vi "FPGAmain.vi"() -> ()   [LabVIEW 2013]
uses:
  FPGA/DataMode.ctl
  FPGA/AcquireState.ctl
  <vilib>/Platform/TimedLoop/XDataNode/timing_clust.ctl
  <vilib>/Platform/TimedLoop/XDataNode/nitl_modes.ctl
  <vilib>/Platform/TimedLoop/XDataNode/wakeup.ctl
  <vilib>/rvi/Emulation/niFpgaSctlEmulationGetInTimedLoop.vi
  <vilib>/rvi/Emulation/niFpgaEmulationReportErrorSimple.vi
  <vilib>/rvi/Emulation/niFpgaGetClockAttributes.vi
  <vilib>/rvi/Emulation/niFpgaCriticalErrorInLSC.vi
  <vilib>/rvi/FIFO/Fifo_Resource/nirvififoEmulationWriteFpgaImpl.vi
  <vilib>/rvi/DataTransferAndStorage/Container/Common/niFpgaContainerGetUniqueNameForEmu.vi
  <vilib>/rvi/FIFO/Fifo_Resource/nirvififoEmulationReadFpgaImpl.vi
  <vilib>/rvi/interface/RandomDataEmulation/nirviRandomDataMultiElementFPGAFIFO.vi
  <instcachedir>/0/nirviRandomDataMultiElementFPGAFIFO_F2B80EDE0D7944A08478D8D26097D4DB.lvgen/nirviRandomDataMultiElementFPGAFIFO_F2B80EDE0D7944A08478D8D26097D4DB_005.vi
  <vilib>/rvi/interface/RandomDataEmulation/niFpgaRandomDataHandleErrors.vi
  <vilib>/rvi/interface/RandomDataEmulation/nirviRandomDataFPGAFIFO.vi
  <vilib>/rvi/eio/common/nirviEmuTemplateMethod_errors.vi
  <vilib>/Platform/TimedLoop/XDataNode/XDataNode.xnode
  <vilib>/rvi/DataTransferAndStorage/Container/XNode/niFpgaContainer.xnode
  <vilib>/rvi/FIFO/Fifo_Resource/nirvififoEmulationWrite.vi
  <vilib>/rvi/FIFO/Fifo_Resource/nirvififoEmulationRead.vi
  <vilib>/rvi/interface/RandomDataEmulation/nirviRandomDataFpgaMultiElementTemplate.vi
  <vilib>/rvi/interface/RandomDataEmulation/nirviRandomDataFpgaReadWriteTemplate.vi
  <vilib>/eio/EIONode/EIONode.xnode
  <vilib>/rvi/FIFO/Fifo_Resource/nirvififoEmulationP2P.vi
  <vilib>/Platform/TimedLoop/XDataNode/XDNodeRunTimeDep.lvlib
  <instrlib>/FlexRIO/Libraries/Helper VIs/NI FlexRIO Helper VIs.lvlib
panel:
  in  "CIC Gain":fxp<+/-,32,1>=0.00390625 format="%#_32g"
  in  "Set downsample":bool
  in  "FIR coeffs":fxp<+/-,18,18>[](array[numeric])
  in  "FIR shift":i32
  in  "new coeffs":bool
  in  "enable filter":bool
  in  "Downsample":fxp<+,8,8>
  in  "Samples Per Trigger":i32 min=1 step=1
  in  "Trigger simulated data":bool
  in  "simulated phase 51600":fxp<+,64,64>
  in  "phase 5160":fxp<+,64,64>
  in  "Simulated phase 5772":fxp<+,64,64>[](array[numeric])=[0.0, 0.0, 0.0, 0.0]
  in  "Mode":T1
  in  "Phase 5772":fxp<+,64,64>[](array[numeric])=[0.0, 0.0, 0.0, 0.0]
  in  "Acquisition running":bool
  in  "User Command Commit":bool
  in  "User Command":u8
  out "User Command Idle":bool
  out "User Command Status":u8
  in  "User Data 0":u16
  in  "User Data 1":u8
  out "PLL Locked":bool
  out "User Error":bool
  out "Configured?":bool
  # "Dynamic filter"
  # "Dynamic downsample"
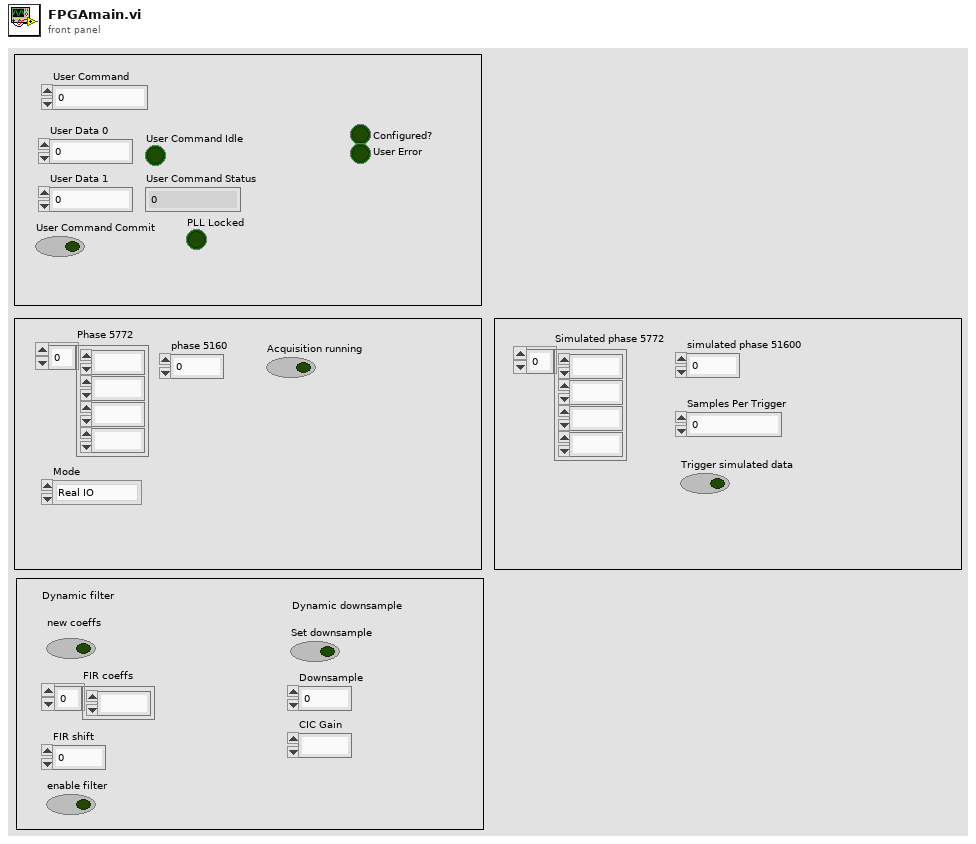
[diagram p1: front panel]
types:
  T1 = typedef "DataMode.ctl" = enum16{"Real IO", "Simulated"}
  T2 = typedef "AcquireState.ctl" = enum8{"Idle", "Acquire"}
  T3 = typedef "XDNodeRunTimeDep.lvlib/timing_clust.ctl" = cluster{"Expected End [f-1]":u64, "Actual End [f-1]":u64, "Finished Late? [f-1]":bool, "Expected End [i-1]":u64, "Actual End [i-1]":u64, "Finished Late? [i-1]":bool, "Expected Start [i]":u64, "Actual Start [i]":u64, "Expected Start [f]":u64, "Actual Start [f]":u64, "Source Name":string, "Structure Name":string, "Period":i64, "Deadline":i64, "Offset":i64, "Start":i64, "Priority":i32, "Timeout":i32, "Mode":T4, "Wakeup Reason":T5, "Error":errorcluster, "Source Type":string, "Secondary Source Type":string, "Global End Time":u64, "Global Start Time":u64, "Frame Duration":u64, "Iteration Duration":u64, "Assigned CPU":i32, "I/O Scan Engine Mode":u32}
  T4 = typedef "XDNodeRunTimeDep.lvlib/nitl_modes.ctl" = enum32{"No Change", "Process missed periods, maintain original phase", "Discard missed periods, maintain original phase", "Process missed periods, ignore original phase", "Discard missed periods, ignore original phase"}
  T5 = typedef "XDNodeRunTimeDep.lvlib/wakeup.ctl" = enum32{"Normal", "Aborted", "Asynchronous wakeup", "Timing source error", "Timed loop error", "Timeout"}
  T6 = typedef "I16 array size 4.ctl" = i16[]
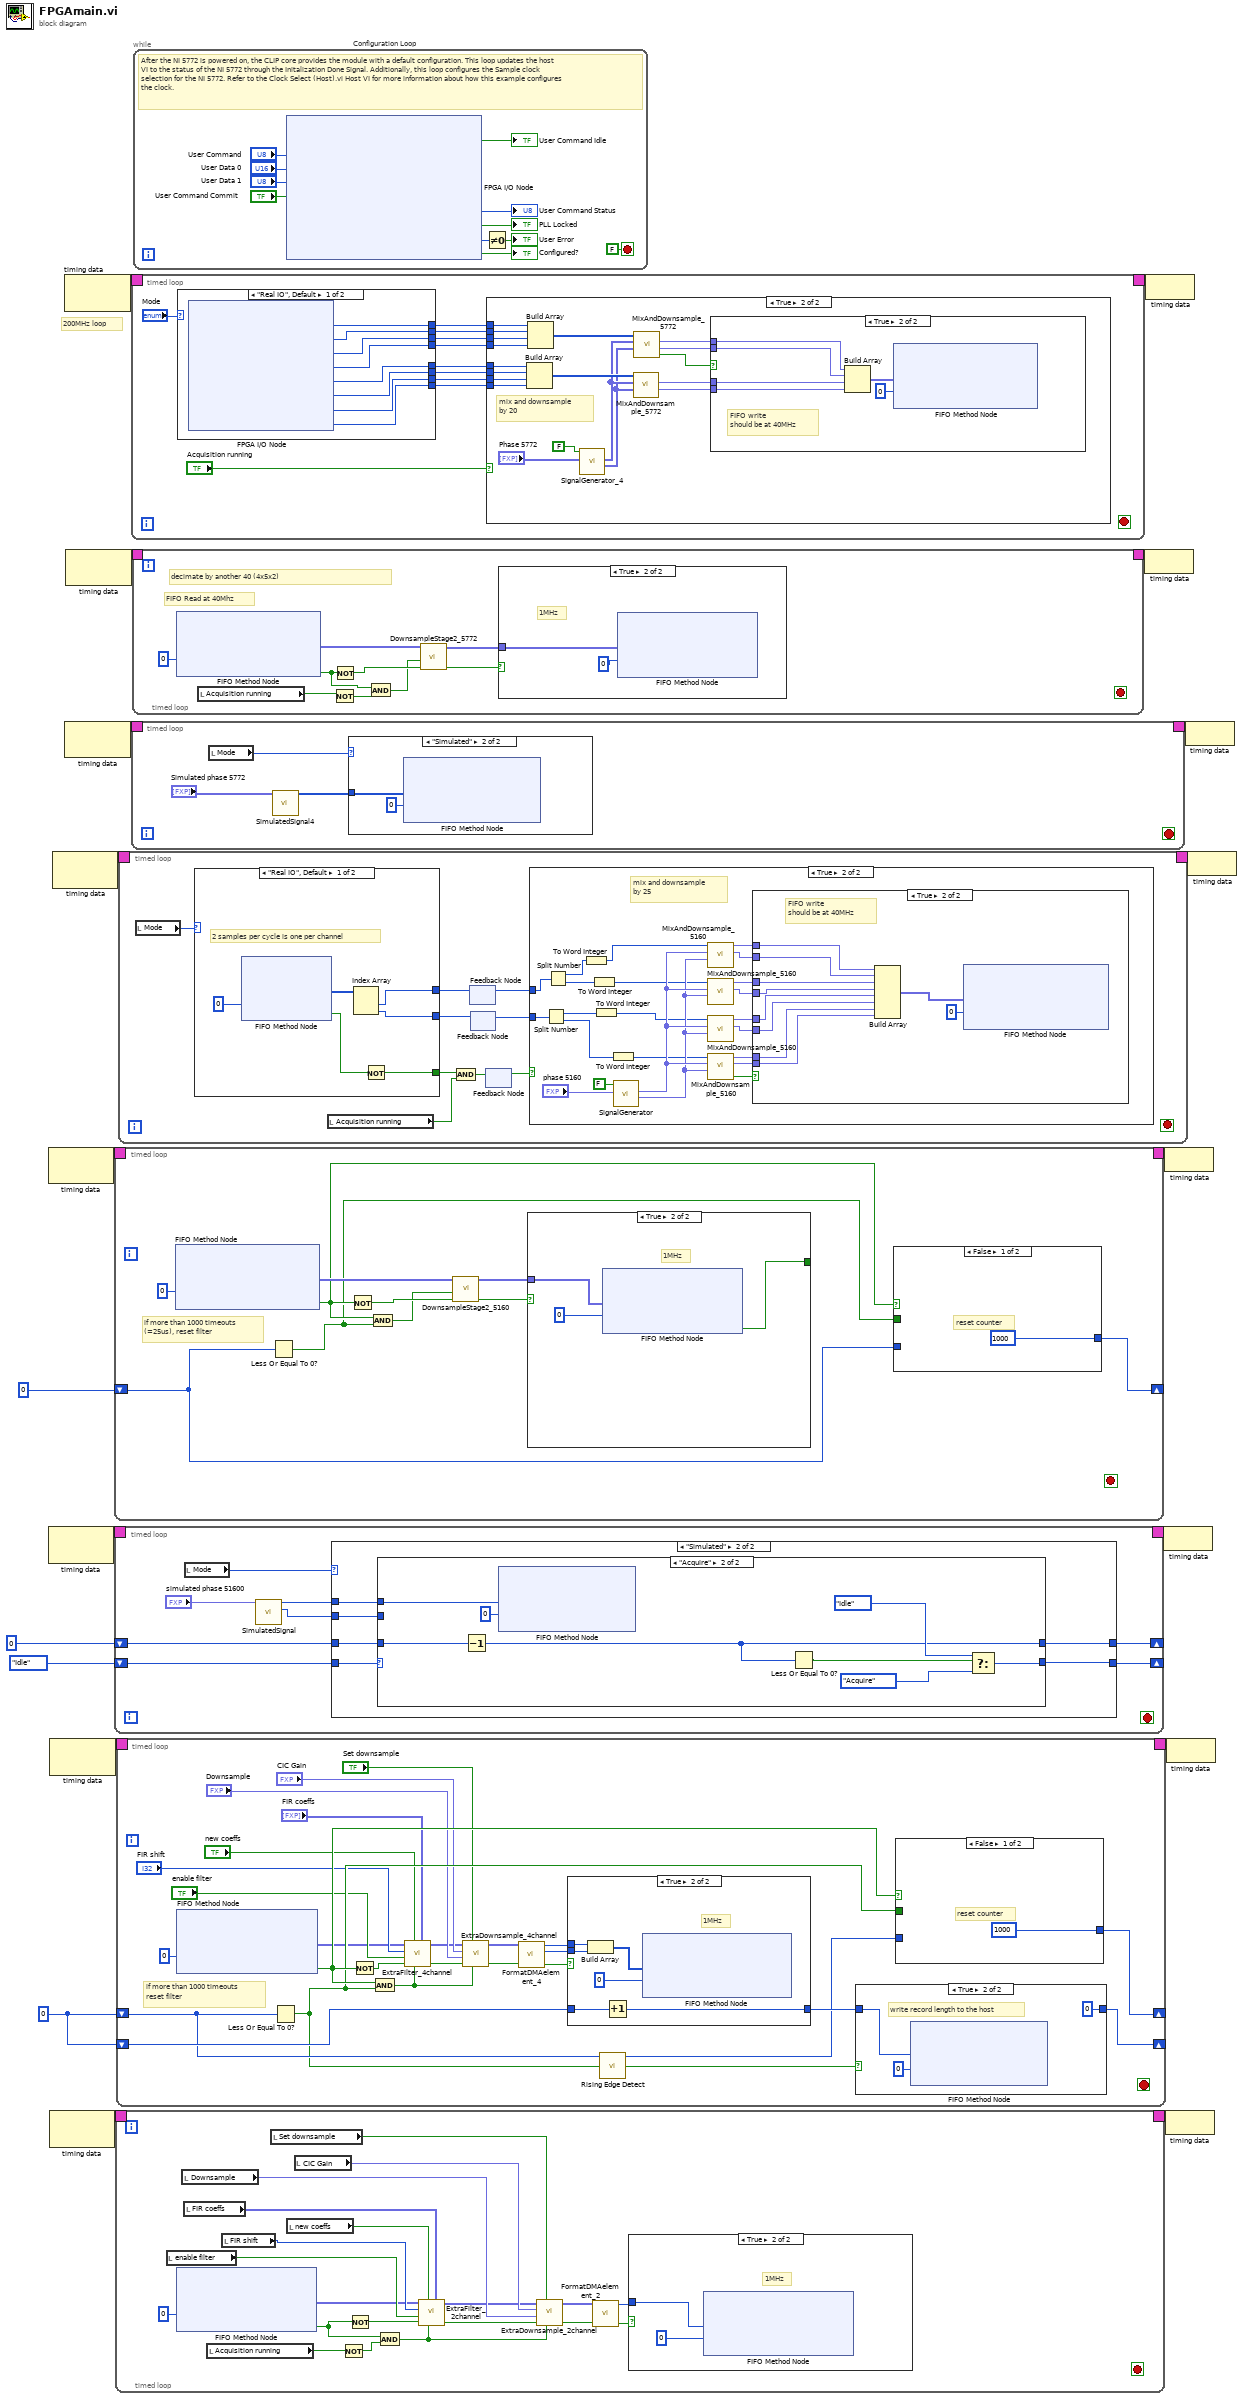
[diagram p0: block diagram]
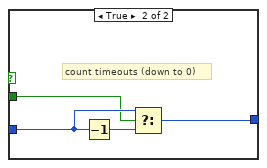
[diagram p3: hidden frame]
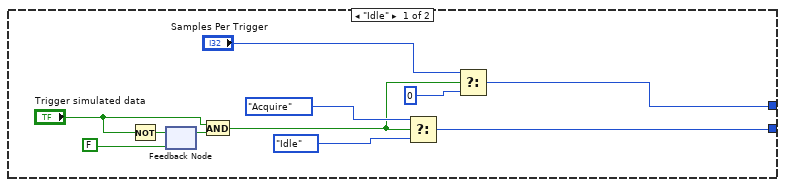
[diagram p7: hidden frame]
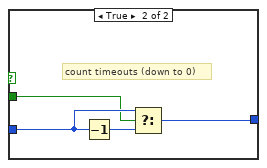
[diagram p8: hidden frame]
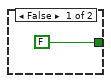
[diagram p9: hidden frame]
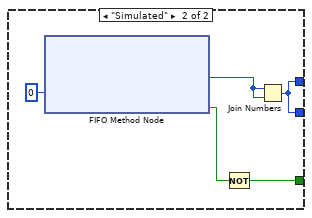
[diagram p12: hidden frame]
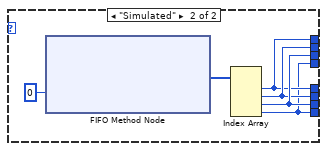
[diagram p17: hidden frame]
diagram:
  w1 = 0 ("y")
  # "200MHz loop"
  n1 = node-c288() -> (w12:T3)  [unwired: 1 in]
  n2 = node-c288() -> (w10:T3)  [unwired: 1 in]
  n3 = node-c288() -> (w3:T3)  [unwired: 1 in]
  n4 = node-c288() -> (w5:T3)  [unwired: 1 in]
  n5 = node-c288() -> (w14:T3)  [unwired: 1 in]
  n6 = node-c288() -> (w20:T3)  [unwired: 1 in]
  n7 = node-c288() -> (w16:T3)  [unwired: 1 in]
  n8 = node-c288() -> (w18:T3)  [unwired: 1 in]
  n9 = timed-loop {
    timing: w12 -> [_]
    timing-out: [_] -> w11
    shift-right: [w23] -> _
    shift-left: 0 ("y") -> [w22]
    stop <- _ stop-if-true
    # "if more than 1000 timeouts\n(=25us), reset filter"
    n10 = xnode ("FIFO Method Node")("Timeout"=0) -> ("Element"=w27:fxp<+/-,16,14>[], "Timed Out?"=w24:bool)  [unwired: 1 in, 1 out]
    n11 = Less Or Equal To 0?(x=w22) -> (x <= 0?=w21:bool)
    n12 = Not(x=w24) -> (.not. x?=w28:bool)
    n13 = And(x=w24, y=w21) -> (x .and. y?=w25:bool)
    n14 = call "DownsampleStage2_5160.vi"("valid in"=w28, "reset"=w25, "Element"=w27) -> ("valid out"=w29:bool, "Array"=w30:fxp<+/-,16,14>[])  [unwired: 7 in]
    n15 = case shown="True" w29 {
      tunnel: w30 -> [_ w37]
      tunnel: [FALSE ("Timed Out?") w38] -> _
      frame False {
      }
      frame True {
        # "1MHz"
        n16 = xnode ("FIFO Method Node")("Element"=w37, "Timeout"=0) -> ("Timed Out?"=w38:bool)  [unwired: 1 in, 1 out]
      }
    }
    n17 = case shown="False" w24 {
      tunnel: w21 -> [_ w33]
      tunnel: w22 -> [_ w34]
      tunnel: [1000 ("y") w32] -> w23
      frame False {
        # "reset counter"
      }
      frame True {
        # "count timeouts (down to 0)"
        n18 = Decrement(x=w34) -> (x-1=w35:i32)
        n19 = Select(t=w34, s=w33, f=w35) -> (s? t:f=w32:i32)
      }
    }
  }
  n20 = timed-loop {
    timing: w10 -> [_]
    timing-out: [_] -> w9
    shift-right: [w45] -> _
    shift-left: 0 ("f") -> [w44]
    shift-right: [w43] -> _
    shift-left: AcquireState."Idle" ("Acquire State") -> [w42]
    stop <- _ stop-if-true
    n21 = local read "Mode"() -> (w49:T1)
    n22 = call "SimulatedSignal.vi"("phase"="simulated phase 51600") -> ("cos output"=w47:i16, "Sample output"=w48:i16)  [unwired: 9 in]
    n23 = case shown="\"Simulated\"" w49 {
      tunnel: w48 -> [_ w57]
      tunnel: w47 -> [_ w52]
      tunnel: [w51 w56] -> w45
      tunnel: w44 -> [w51 w55]
      tunnel: [w50 w54] -> w43
      tunnel: w42 -> [w50 w53]
      frame "Real IO" {
      }
      frame "Simulated" {
        n24 = case shown="\"Acquire\"" w53 {
          tunnel: w55 -> [_ w73]
          tunnel: [w62 w72] -> w54
          tunnel: [w59 w71] -> w56
          tunnel: w57 -> [_ w70]
          tunnel: w52 -> [_ _]
          frame "Idle" {
            n25 = Not(x="Trigger simulated data") -> (.not. x?=w63:bool)
            n26 = feedback #1(FALSE) -> (w64:bool)
            n27 = feedback-in #1(w63) -> ()
            n28 = And(x="Trigger simulated data", y=w64) -> (x .and. y?=w58:bool)
            n29 = Select(t=AcquireState."Acquire" ("Acquire State"), s=w58, f=AcquireState."Idle" ("Acquire State")) -> (s? t:f=w62:T2)
            n30 = Select(t="Samples Per Trigger", s=w58, f=0) -> (s? t:f=w59:i32)
          }
          frame "Acquire" {
            n31 = Decrement(x=w73) -> (x-1=w71:i32)
            n32 = xnode ("FIFO Method Node")("Element"=w70, "Timeout"=0) -> ()  [unwired: 1 in, 2 out]
            n33 = Less Or Equal To 0?(x=w71) -> (x <= 0?=w75:bool)
            n34 = Select(t=AcquireState."Idle" ("Acquire State"), s=w75, f=AcquireState."Acquire" ("Acquire State")) -> (s? t:f=w72:T2)
          }
        }
      }
    }
  }
  n35 = timed-loop {
    timing: w3 -> [_]
    timing-out: [_] -> w2
    stop <- _ stop-if-true
    n36 = local read "enable filter"() -> (w94:bool)
    n37 = xnode ("FIFO Method Node")("Timeout"=0) -> ("Element"=w85:fxp<+/-,16,14>[], "Timed Out?"=w89:bool)  [unwired: 1 in, 1 out]
    n38 = local read "Downsample"() -> (w93:fxp<+,8,8>)
    n39 = local read "FIR coeffs"() -> (w97:fxp<+/-,18,18>[])
    n40 = local read "Acquisition running"() -> (w91:bool)
    n41 = local read "FIR shift"() -> (w95:i32)
    n42 = local read "Set downsample"() -> (w92:bool)
    n43 = local read "new coeffs"() -> (w96:bool)
    n44 = local read "CIC Gain"() -> (w87:fxp<+/-,32,1>)
    n45 = Not(x=w91) -> (.not. x?=w90:bool)
    n46 = Not(x=w89) -> (.not. x?=w84:bool)
    n47 = And(x=w89, y=w90) -> (x .and. y?=w88:bool)
    n48 = call "ExtraFilter_2channel.vi"(5:"new coeffs"=w97, "reset"=w88, 7:"new coeffs"=w96, "valid in"=w84, "enable filter"=w94, "new shift"=w95, "Data in"=w85) -> ("valid out"=w83:bool, "Data out"=w86:fxp<+/-,16,14>[])  [unwired: 3 in]
    n49 = call "ExtraDownsample_2channel.vi"("reset"=w88, "Set downsample"=w92, "valid in"=w83, "Downsample"=w93, "CIC Gain"=w87, "Data in"=w86) -> ("valid out"=w80:bool, "Data out"=w82:fxp<+/-,16,14>[])  [unwired: 4 in]
    n50 = call "FormatDMAelement_2.vi"("valid in"=w80, "Data in"=w82) -> ("valid out"=w79:bool, "Element1"=w81:u64)  [unwired: 8 in]
    n51 = case shown="True" w79 {
      tunnel: w81 -> [_ w99]
      frame False {
      }
      frame True {
        # "1MHz"
        n52 = xnode ("FIFO Method Node")("Element"=w99, "Timeout"=0) -> ()  [unwired: 1 in, 2 out]
      }
    }
  }
  n53 = timed-loop {
    timing: w5 -> [_]
    timing-out: [_] -> w4
    shift-right: [w123] -> _
    shift-left: w1 -> [w122]
    shift-right: [w125] -> _
    shift-left: w1 -> [w127]
    stop <- _ stop-if-true
    # "if more than 1000 timeouts\nreset filter"
    n54 = xnode ("FIFO Method Node")("Timeout"=0) -> ("Element"=w111:fxp<+/-,16,14>[], "Timed Out?"=w124:bool)  [unwired: 1 in, 1 out]
    n55 = Less Or Equal To 0?(x=w122) -> (x <= 0?=w121:bool)
    n56 = Not(x=w124) -> (.not. x?=w109:bool)
    n57 = And(x=w124, y=w121) -> (x .and. y?=w119:bool)
    n58 = call "ExtraFilter_4channel.vi"(5:"new coeffs"="FIR coeffs", "reset"=w119, 7:"new coeffs"="new coeffs", "valid in"=w109, "enable filter"="enable filter", "new shift"="FIR shift", "Data in"=w111) -> ("valid out"=w108:bool, "Data out"=w110:fxp<+/-,16,14>[])  [unwired: 3 in]
    n59 = call "ExtraDownsample_4channel.vi"("reset"=w119, "Set downsample"="Set downsample", "valid in"=w108, "Downsample"="Downsample", "CIC Gain"="CIC Gain", "Data in"=w110) -> ("valid out"=w104:bool, "Data out"=w107:fxp<+/-,16,14>[])  [unwired: 4 in]
    n60 = call "FormatDMAelement_4.vi"("valid in"=w104, "Data in"=w107) -> ("valid out"=w103:bool, "Element2"=w105:u64, "Element1"=w106:u64)  [unwired: 7 in]
    n61 = case shown="True" w103 {
      tunnel: w106 -> [_ w143]
      tunnel: w105 -> [_ w142]
      tunnel: w127 -> [w138 w140]
      tunnel: [w138 w139] -> w126
      frame False {
      }
      frame True {
        # "1MHz"
        n62 = Build Array(w143, w142) -> (w141:u64[])
        n63 = Increment(x=w140) -> (x+1=w139:i32)
        n64 = xnode ("FIFO Method Node")("Element"=w141, "Timeout"=0) -> ()  [unwired: 1 in, 2 out]
      }
    }
    n65 = call <instrlib>:"Rising Edge Detect.vi"("signal"=w121) -> ("edge detected"=w120:bool)  [unwired: 14 in]
    n66 = case shown="True" w120 {
      tunnel: w126 -> [w134 w135]
      tunnel: [w134 0 ("y")] -> w125
      frame False {
      }
      frame True {
        # "write record length to the host"
        n67 = xnode ("FIFO Method Node")("Element"=w135, "Timeout"=0) -> ()  [unwired: 1 in, 2 out]
      }
    }
    n68 = case shown="False" w124 {
      tunnel: w121 -> [_ w131]
      tunnel: w122 -> [_ w132]
      tunnel: [1000 ("y") w130] -> w123
      frame False {
        # "reset counter"
      }
      frame True {
        # "count timeouts (down to 0)"
        n69 = Decrement(x=w132) -> (x-1=w133:i32)
        n70 = Select(t=w132, s=w131, f=w133) -> (s? t:f=w130:i32)
      }
    }
  }
  n71 = timed-loop {
    timing: w14 -> [_]
    timing-out: [_] -> w13
    stop <- _ stop-if-true
    n72 = local read "Mode"() -> (w150:T1)
    n73 = case shown="\"Real IO\", Default" w150 {
      tunnel: [w192 w198] -> w155
      tunnel: [w189 w195] -> w149
      tunnel: [w191 w198] -> w152
      frame "Real IO", Default {
        # "2 samples per cycle is one per channel"
        n74 = xnode ("FIFO Method Node")("Timeout"=0) -> ("Element"=w194:u32[], "Timed Out?"=w190:bool)  [unwired: 1 in, 1 out]
        n75 = Index Array(array=w194) -> (element #1=w192:u32, element #2=w191:u32)  [unwired: 2 in]
        n76 = Not(x=w190) -> (.not. x?=w189:bool)
      }
      frame "Simulated" {
        n77 = xnode ("FIFO Method Node")("Timeout"=0) -> ("Element"=w197:i16, "Timed Out?"=w196:bool)  [unwired: 1 in, 1 out]
        n78 = Not(x=w196) -> (.not. x?=w195:bool)
        n79 = Join Numbers(hi=w197, lo=w197) -> ((hi.lo)=w198:u32)
      }
    }
    n80 = local read "Acquisition running"() -> (w148:bool)
    n81 = And(x=w149, y=w148) -> (x .and. y?=w147:bool)
    n82 = feedback-in #2(w155) -> ()
    n83 = feedback #2() -> (w154:u32)  [unwired: 1 in]
    n84 = feedback #3() -> (w151:u32)  [unwired: 1 in]
    n85 = feedback-in #3(w152) -> ()
    n86 = feedback #4() -> (w153:bool)  [unwired: 1 in]
    n87 = feedback-in #4(w147) -> ()
    n88 = case shown="True" w153 {
      tunnel: w154 -> [_ w169]
      tunnel: w151 -> [_ w158]
      frame False {
        # "FIFO read timeout, no data"
      }
      frame True {
        # "mix and downsample\nby 25"
        n89 = Split Number(x=w158) -> (hi(x)=w159:u16, lo(x)=w160:u16)
        n90 = Split Number(x=w169) -> (hi(x)=w168:u16, lo(x)=w167:u16)
        n91 = To Word Integer(number=w168) -> (16bit integer=w162:i16)
        n92 = To Word Integer(number=w167) -> (16bit integer=w161:i16)
        n93 = To Word Integer(number=w159) -> (16bit integer=w156:i16)
        n94 = To Word Integer(number=w160) -> (16bit integer=w157:i16)
        n95 = call "SignalGenerator.vi"("phase"="phase 5160", "Reset"=FALSE) -> ("Cos"=w163:fxp<+/-,16,0>, "Sin"=w164:fxp<+/-,16,0>)  [unwired: 7 in, 1 out]
        n96 = call "MixAndDownsample_5160.vi"("Sine in"=w163, "Cosine in"=w164, "Sample in"=w162) -> ("Q out"=w176:fxp<+/-,16,14>, "I out"=w178:fxp<+/-,16,14>)  [unwired: 6 in, 1 out]
        n97 = call "MixAndDownsample_5160.vi"("Sine in"=w163, "Cosine in"=w164, "Sample in"=w161) -> ("Q out"=w174:fxp<+/-,16,14>, "I out"=w175:fxp<+/-,16,14>)  [unwired: 6 in, 1 out]
        n98 = call "MixAndDownsample_5160.vi"("Sine in"=w163, "Cosine in"=w164, "Sample in"=w156) -> ("Q out"=w172:fxp<+/-,16,14>, "I out"=w173:fxp<+/-,16,14>)  [unwired: 6 in, 1 out]
        n99 = call "MixAndDownsample_5160.vi"("Sine in"=w163, "Cosine in"=w164, "Sample in"=w157) -> ("valid out"=w177:bool, "Q out"=w170:fxp<+/-,16,14>, "I out"=w171:fxp<+/-,16,14>)  [unwired: 6 in]
        n100 = case shown="True" w177 {
          tunnel: w178 -> [_ w187]
          tunnel: w176 -> [_ w186]
          tunnel: w175 -> [_ w185]
          tunnel: w174 -> [_ w179]
          tunnel: w173 -> [_ w184]
          tunnel: w172 -> [_ w183]
          tunnel: w171 -> [_ w182]
          tunnel: w170 -> [_ w181]
          frame False {
          }
          frame True {
            # "FIFO write\nshould be at 40MHz"
            n101 = Build Array(w187, w186, w185, w179, w184, w183, w182, w181) -> (w180:fxp<+/-,16,14>[])
            n102 = xnode ("FIFO Method Node")("Element"=w180, "Timeout"=0) -> ()  [unwired: 1 in, 2 out]
          }
        }
      }
    }
  }
  n103 = timed-loop {
    timing: w20 -> [_]
    timing-out: [_] -> w19
    stop <- _ stop-if-true
    n104 = case shown="\"Real IO\", Default" "Mode" {
      tunnel: [w244 w246] -> w211
      tunnel: [w243 w247] -> w210
      tunnel: [w237 w248] -> w209
      tunnel: [w242 w245] -> w208
      tunnel: [w241 w246] -> w206
      tunnel: [w240 w247] -> w205
      tunnel: [w239 w245] -> w204
      tunnel: [w238 w248] -> w203
      frame "Real IO", Default {
        n105 = xnode "FPGA I/O Node"() -> ("IO Module\\AI 0 Data N-3"=w244:i16, "IO Module\\AI 0 Data N-2"=w243:i16, "IO Module\\AI 0 Data N-1"=w237:i16, "IO Module\\AI 0 Data N"=w242:i16, "IO Module\\AI 1 Data N-3"=w241:i16, "IO Module\\AI 1 Data N-2"=w240:i16, "IO Module\\AI 1 Data N-1"=w238:i16, "IO Module\\AI 1 Data N"=w239:i16)  [unwired: 8 in, 8 out]
      }
      frame "Simulated" {
        n106 = xnode ("FIFO Method Node")("Timeout"=0) -> ("Element"=w249:i16[])  [unwired: 1 in, 2 out]
        n107 = Index Array(array=w249) -> (element #1=w246:i16, element #2=w247:i16, element #3=w248:i16, element #4=w245:i16)  [unwired: 4 in]
      }
    }
    n108 = case shown="True" "Acquisition running" {
      tunnel: w211 -> [_ w230]
      tunnel: w210 -> [_ w229]
      tunnel: w209 -> [_ w228]
      tunnel: w208 -> [_ w227]
      tunnel: w206 -> [_ w226]
      tunnel: w205 -> [_ w225]
      tunnel: w204 -> [_ w224]
      tunnel: w203 -> [_ w223]
      frame False {
      }
      frame True {
        # "mix and downsample\nby 20"
        n109 = Build Array(w226, w225, w223, w224) -> (w221:i16[])
        n110 = Build Array(w230, w229, w228, w227) -> (w222:i16[])
        n111 = call "SignalGenerator_4.vi"("Phase"="Phase 5772", "reset"=FALSE) -> ("Sine out"=w213:fxp<+/-,16,0>[], "Cosine out"=w214:fxp<+/-,16,0>[])  [unwired: 8 in]
        n112 = call "MixAndDownsample_5772.vi"("Sine in"=w213, "Cosine in"=w214, "Signal Input"=w221) -> ("Q out"=w216:fxp<+/-,16,14>, "I out"=w217:fxp<+/-,16,14>)  [unwired: 6 in, 1 out]
        n113 = call "MixAndDownsample_5772.vi"("Sine in"=w213, "Cosine in"=w214, "Signal Input"=w222) -> ("data valid"=w218:bool, "Q out"=w219:fxp<+/-,16,14>, "I out"=w220:fxp<+/-,16,14>)  [unwired: 6 in]
        n114 = case shown="True" w218 {
          tunnel: w219 -> [_ w236]
          tunnel: w220 -> [_ w233]
          tunnel: w217 -> [_ w232]
          tunnel: w216 -> [_ w231]
          frame False {
          }
          frame True {
            # "FIFO write\nshould be at 40MHz"
            n115 = Build Array(w233, w236, w232, w231) -> (w235:fxp<+/-,16,14>[])
            n116 = xnode ("FIFO Method Node")("Element"=w235, "Timeout"=0) -> ()  [unwired: 1 in, 2 out]
          }
        }
      }
    }
  }
  n117 = timed-loop {
    timing: w16 -> [_]
    timing-out: [_] -> w15
    stop <- _ stop-if-true
    n118 = local read "Mode"() -> (w255:T1)
    n119 = call "SimulatedSignal4.vi"("Phase"="Simulated phase 5772") -> ("output"=w254:T6)  [unwired: 9 in, 1 out]
    n120 = case shown="\"Simulated\"" w255 {
      tunnel: w254 -> [_ w256]
      frame "Real IO", Default {
      }
      frame "Simulated" {
        n121 = xnode ("FIFO Method Node")("Element"=w256, "Timeout"=0) -> ()  [unwired: 1 in, 2 out]
      }
    }
  }
  n122 = timed-loop {
    timing: w18 -> [_]
    timing-out: [_] -> w17
    stop <- _ stop-if-true
    # "FIFO Read at 40Mhz"
    # "decimate by another 40 (4x5x2)"
    n123 = xnode ("FIFO Method Node")("Timeout"=0) -> ("Element"=w267:fxp<+/-,16,14>[], "Timed Out?"=w262:bool)  [unwired: 1 in, 1 out]
    n124 = local read "Acquisition running"() -> (w263:bool)
    n125 = Not(x=w263) -> (.not. x?=w261:bool)
    n126 = Not(x=w262) -> (.not. x?=w266:bool)
    n127 = And(x=w262, y=w261) -> (x .and. y?=w260:bool)
    n128 = call "DownsampleStage2_5772.vi"("valid in"=w266, "reset"=w260, "Data in"=w267) -> ("valid out"=w264:bool, "data out"=w265:fxp<+/-,16,14>[])  [unwired: 7 in]
    n129 = case shown="True" w264 {
      tunnel: w265 -> [_ w269]
      frame False {
      }
      frame True {
        # "1MHz"
        n130 = xnode ("FIFO Method Node")("Element"=w269, "Timeout"=0) -> ()  [unwired: 1 in, 2 out]
      }
    }
  }
  n131 = while "Configuration Loop" {
    stop <- FALSE stop-if-true
    # "After the NI 5772 is powered on, the CLIP core provides the module with a default configuration. This loop updates the host VI to the status of the NI 5772 through the Initalization Done Signal. Additionally, this loop configures the Sample clock selection for the NI 5772. Refer to the Clock Select (Host).vi Host VI for more information about how this example configures the clock."
    n132 = xnode "FPGA I/O Node"("IO Module\\User Command"="User Command", "IO Module\\User Data 0"="User Data 0", "IO Module\\User Data 1"="User Data 1", "IO Module\\User Command Commit"="User Command Commit") -> ("IO Module\\User Command Idle"=→"User Command Idle":bool, "IO Module\\User Command Status"=→"User Command Status":u8, "IO Module\\PLL Locked"=→"PLL Locked":bool, "IO Module\\User Error"=w278:u8, "IO Module\\Initialization Done"=→"Configured?":bool)  [unwired: 9 in, 9 out]
    n133 = Not Equal To 0?(x=w278) -> (x != 0?=→"User Error":bool)
  }
  n134 = node-c288(w17) -> ()
  n135 = node-c288(w19) -> ()
  n136 = node-c288(w9) -> ()
  n137 = node-c288(w11) -> ()
  n138 = node-c288(w2) -> ()
  n139 = node-c288(w4) -> ()
  n140 = node-c288(w15) -> ()
  n141 = node-c288(w13) -> ()
